vi "ExSpectGetGratingType.vi"() -> ()   [LabVIEW 2010]
panel:
  out "Label":string
  out "Grooves":dbl format="%.1f"
  in  "Grating Number":i16=1 min=1 max=6 step=1
  out "error out":errorcluster
  in  "error in (no error)":errorcluster
  # "ExSpectGetGratingType.vi\n(Normal Spectrograph via USB/COM port)\nThis VI will read the current grating Grooves and Label."
  # "NOTES:\nA properly configured spectometer .ini must be present in the LabVIEW folder for spectrograph operation.\n\nConsult the Toolkit documentation for more information on how to configure this file."
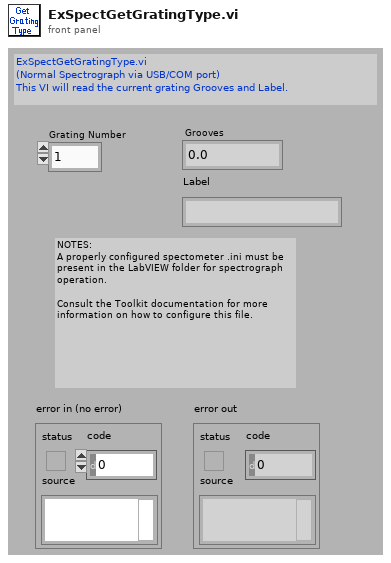
[diagram p1: front panel]
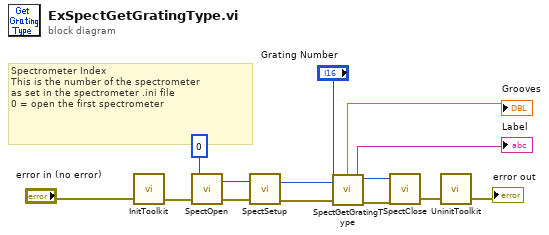
[diagram p0: block diagram]
diagram:
  # "Spectrometer Index\nThis is the number of the spectrometer\nas set in the spectrometer .ini file\n0 = open the first spectrometer"
  n1 = call <userlib>:"InitToolkit.vi"("error in"="error in (no error)") -> ("error out"=w13:errorcluster)
  n2 = call <userlib>:"SpectOpen.vi"("error in"=w13, "Spectrometer ID"=0) -> ("error out"=w12:errorcluster, "Spectrometer Handle"=w8:u32)  [unwired: 1 in]
  n3 = call <userlib>:"SpectSetup.vi"("error in"=w12, "Spectrometer Handle"=w8) -> ("error out"=w7:errorcluster, "Spectrometer Handle"=w5:u32)
  n4 = call <userlib>:"SpectGetGratingType.vi"("Spectrometer Handle"=w5, "Grating Number"="Grating Number", "error in"=w7) -> ("Spectrometer Handle"=w3:u32, "Grooves per mm"=→"Grooves":dbl, "Label"=→"Label":string, "error out"=w6:errorcluster)
  n5 = call <userlib>:"SpectClose.vi"("error in"=w6, "Spectrometer Handle"=w3) -> ("error out"=w11:errorcluster)
  n6 = call <userlib>:"UninitToolkit.vi"("error in"=w11) -> ("error out"=→"error out":errorcluster)
